vi "CheckForError.vi"(8 "Error In":errorcluster, 11 "MainData In":T1={"Image"={"image type"=0, "image depth"=32, "image"=array[640000 elements], "mask"=array[20000 elements], "colors"=[], "Rectangle"={"left"=0, "top"=0, "right"=400, "bottom"=400}}, " TmpImage"={"image type"=0, "image depth"=32, "image"=array[640000 elements], "mask"=array[20000 elements], "colors"=[], "Rectangle"={"left"=0, "top"=0, "right"=400, "bottom"=400}}, "BGColor"=15256322, "FGColor"=13283586, "DRColor"=13283586, "Picture"=bytes[500030], "Queue "=refnum, "EndGameEvent"=refnum, "AnalizeMove"=FALSE}) -> (0 "Error Out":errorcluster)   [LabVIEW 2020]
doc: "Check for erros and passes to handler procedure."
uses:
  typeDef/MainDataCluster.ctl
  <vilib>/picture/picture.llb/imagedata.ctl
  typeDef/StateMachineEnum.ctl
  typeDef/EventData.ctl
  typeDef/EndType.ctl
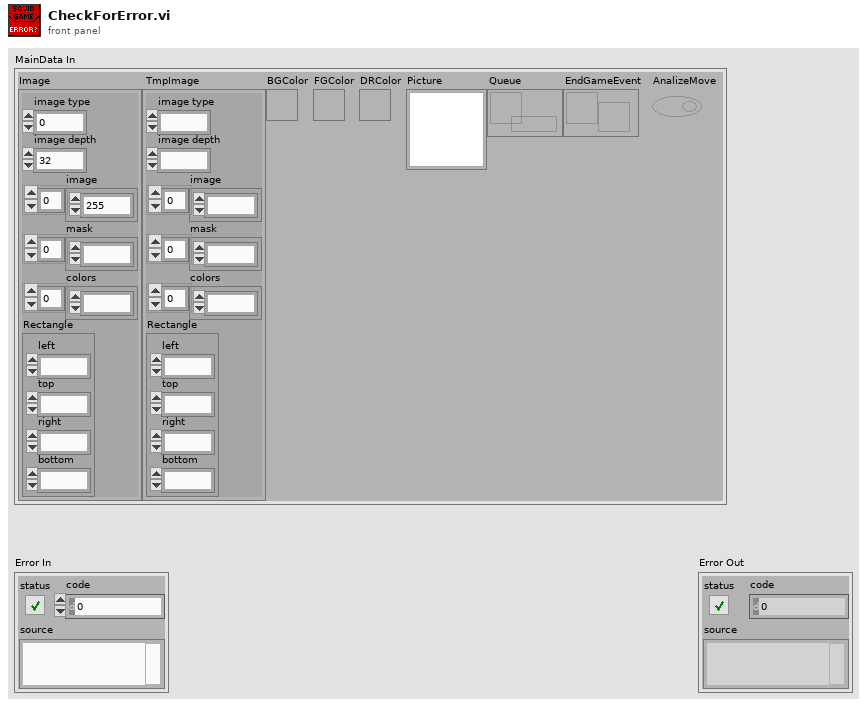
[diagram p1: front panel]
types:
  T1 = typedef "MainDataCluster.ctl" = cluster{"Image":T2, " TmpImage":T2, "BGColor":u32, "FGColor":u32, "DRColor":u32, "Picture":picture, "Queue ":refnum<queue>, "EndGameEvent":refnum<user-event>, "AnalizeMove":bool}
  T2 = typedef "imagedata.ctl" = cluster{"image type":i32, "image depth":i32, "image":u8[], "mask":u8[], "colors":u32[], "Rectangle":cluster{"left":i16, "top":i16, "right":i16, "bottom":i16}}
  T3 = typedef "StateMachineEnum.ctl" = enum16{"Init", "ReadTime", "StartTimer", "Result", "StopTimer", "ErrorHandler", "Close"}
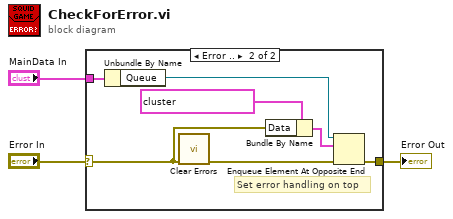
[diagram p0: block diagram]
diagram:
  n1 = case shown="Error .." "Error In" {
    selector: "Error In" -> [w4 w7]
    tunnel: [w4 w5] -> w2
    tunnel: "MainData In" -> [_ w11]
    frame No Error {
    }
    frame Error {
      # "Set error handling on top"
      n2 = Unbundle By Name(w11) -> ("Queue"=w10:refnum<queue>)
      n3 = call <vilib>:"Clear Errors.vi"("error in (no error)"=w7) -> ("error out"=w6:errorcluster)  [unwired: 5 in, 1 out]
      n4 = Bundle By Name(cluster=cluster{"Data":variant, "State":T3} {"Data"=variant, "State"=enum."ErrorHandler"} ("element"), "Data"=w7) -> (w8:cluster{"Data":variant, "State":T3})
      n5 = Enqueue Element At Opposite End(queue=w10, element=w8, error in (no error)=w6) -> (error out=w5:errorcluster)  [unwired: 1 in, 2 out]
    }
  }
  "Error Out" <- w2
